vi "lstsqr_lines.vi"(8 "input error":errorcluster, 9 "weights":dbl[](array[numeric]), 10 "B points":dbl[][](array[numeric])=[[5.0, 3.0], [6.0, 6.0]], 11 "A points":dbl[][](array[numeric])=[[0.0, 1.0], [2.0, 3.0]]) -> (0 "output error":errorcluster, 3 "center":dbl[](array[numeric]))   [LabVIEW 2015]
doc: "This vi finds least square intersection point of lines defined by 2 points in arrays A and B.\nA and B are two-column arrays each containing 1 point coordiantes from each line.\nThe algorithm was adopted from \"Johannes Traa, Least-Squares Intersection of Lines, UIUC 2013\"\n\nINPUT:\nA points - 2xN array of first points that define lines (x,y)\nB points - 2xN array of second points that define lines (x,y)\nweights - 1D array\n\nOUTPUT:\ncenter - calculated least-square center of the intersection of lines\n\nAuthor: Anatolii Kashchuk"
uses:
  <vilib>/Analysis/Matrix/Datatypes/RealMatrix.ctl
  <vilib>/Utility/error.llb/Error Cluster From Error Code.vi
  <vilib>/Analysis/7linalg.llb/Solve Linear Equations (multiple right hand).vi
  <vilib>/Analysis/Matrix/Numeric/Conversions/Matrix To Array - RM.vi
  <vilib>/ErrorRing/Error Ring.xnode
  <vilib>/Analysis/NI_AALPro.lvlib
  <vilib>/Analysis/Matrix/NI_Matrix.lvlib
panel:
  out "Solution Matrix":T1
  out "q":T1
  out "R":T1
  out "XY Graph":cluster{dbl[], dbl[]}[](graph)
  # "Author: Anatolii Kashchuk"
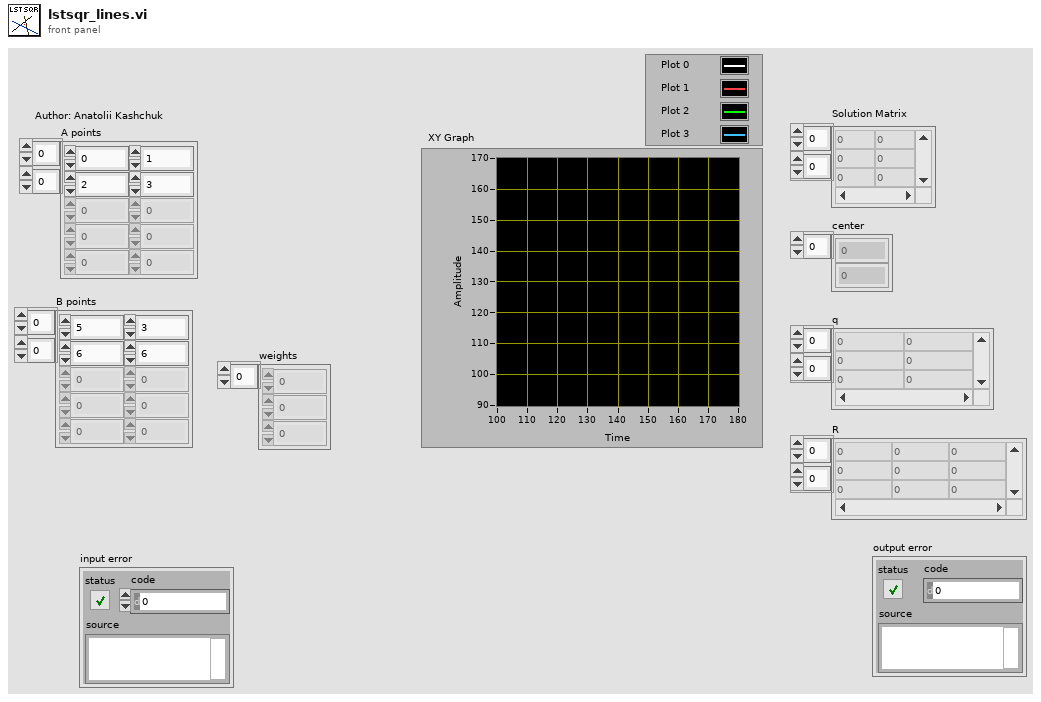
[diagram p1: front panel]
types:
  T1 = typedef "NI_Matrix.lvlib/RealMatrix.ctl" = dbl[][]
  T2 = cluster{"Real 2D Array":dbl[], "Real 2D Array":dbl[]}
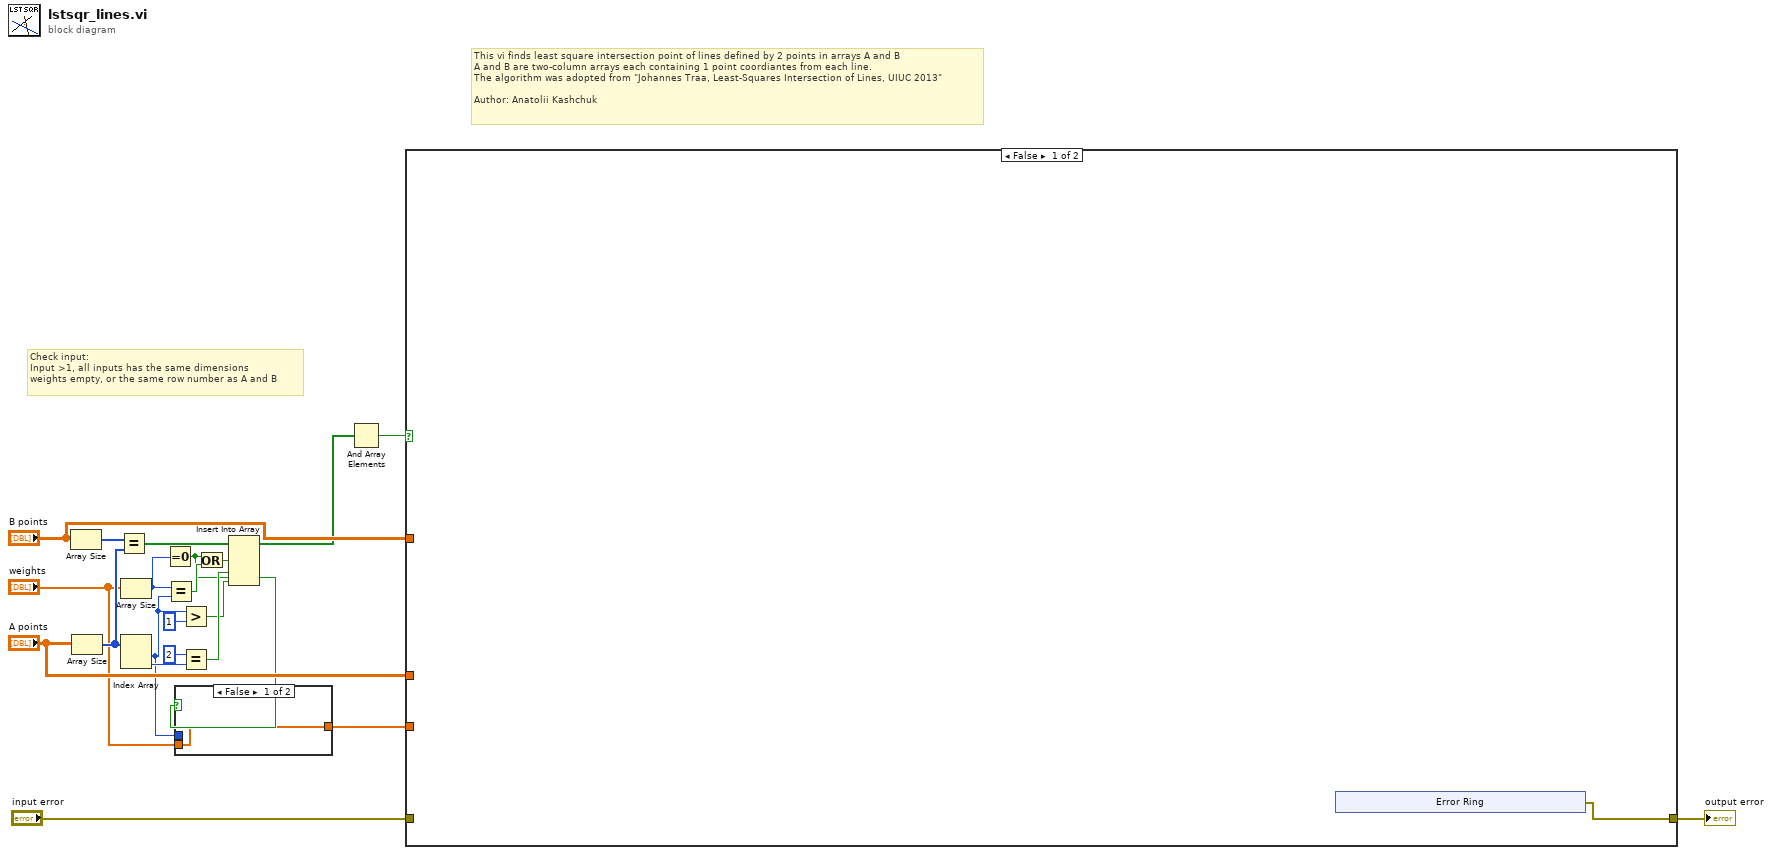
[diagram p0: block diagram]
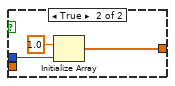
[diagram p2: hidden frame]
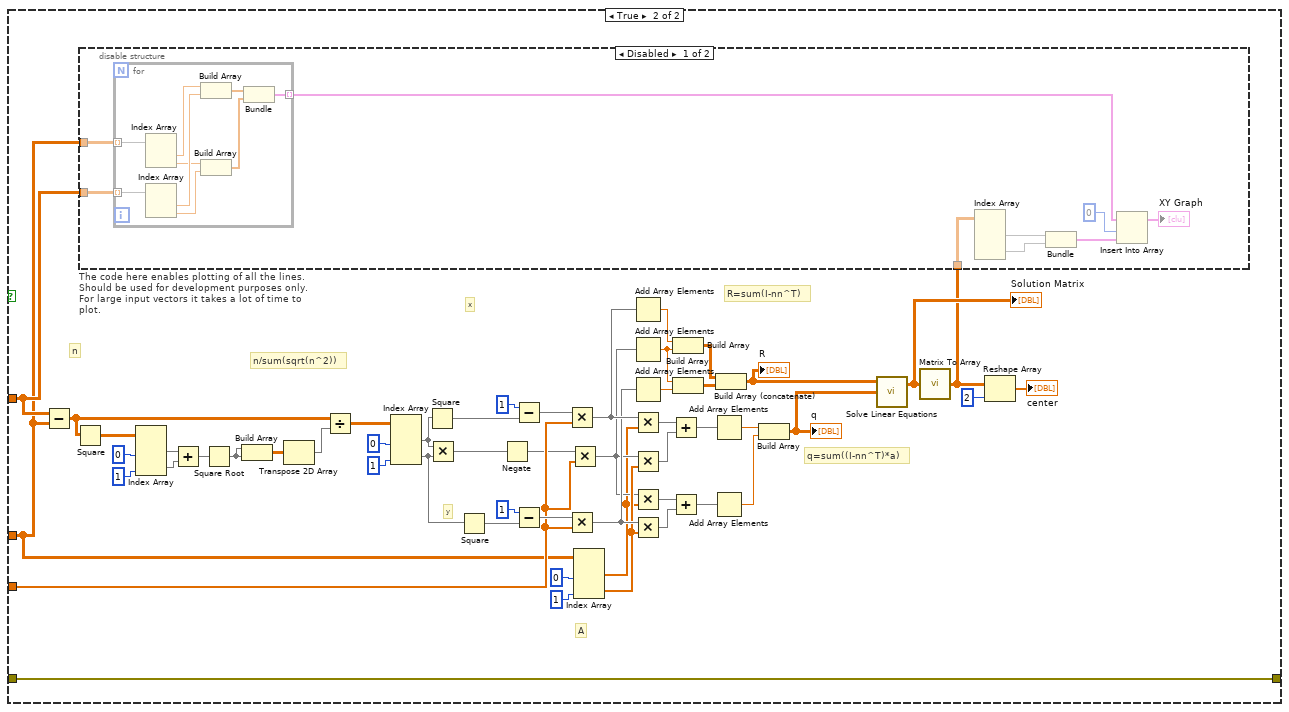
[diagram p3: hidden frame]
diagram:
  # "Check input:\nInput >1, all inputs has the same dimensions\nweights empty, or the same row number as A and B"
  # "This vi finds least square intersection point of lines defined by 2 points in arrays A and B\nA and B are two-column arrays each containing 1 point coordiantes from each line.\nThe algorithm was adopted from \"Johannes Traa, Least-Squares Intersection of Lines, UIUC 2013\"\n\nAuthor: Anatolii Kashchuk"
  n1 = Array Size(array="B points") -> (size(s)=w18:i32[])
  n2 = Array Size(array="A points") -> (size(s)=w17:i32[])
  n3 = Equal?(x=w18, y=w17) -> (x = y?=w14:bool[])
  n4 = Array Size(array="weights") -> (size(s)=w7:i32)
  n5 = Index Array(array=w17) -> (element #1=w4:i32, element #2=w16:i32)  [unwired: 2 in]
  n6 = Equal To 0?(x=w7) -> (x = 0?=w1:bool)
  n7 = Equal?(x=w7, y=w4) -> (x = y?=w6:bool)
  n8 = case shown="False" w1 {
    tunnel: w4 -> [_ w24]
    tunnel: [w22 w23] -> w3
    tunnel: "weights" -> [w22 _]
    frame False {
    }
    frame True {
      n9 = Initialize Array(1.0 ("element"), w24) -> (w23:dbl[])
    }
  }
  n10 = Greater?(x=w4, y=1) -> (0:w11:bool)
  n11 = Equal?(x=2, y=w16) -> (x = y?=w12:bool)
  n12 = Or(x=w1, y=w6) -> (x .or. y?=w5:bool)
  n13 = Insert Into Array(array=w14, new element #1=w5, new element #2=w12, new element #3=w11) -> (w13:bool[])  [unwired: 1 in]
  n14 = And Array Elements(Boolean array=w13) -> (logical AND=w19:bool)
  n15 = case shown="False" w19 {
    tunnel: w3 -> [_ w58]
    tunnel: "A points" -> [_ w49]
    tunnel: "B points" -> [_ w76]
    tunnel: "input error" -> [_ w75]
    tunnel: [w26 w75] -> w8
    frame False {
      n16 = xnode "Error Ring"() -> ("error out"=w26:errorcluster)
    }
    frame True {
      # "A"
      # "n"
      # "y"
      # "x"
      # "q=sum((I-nn^T)*a)"
      # "R=sum(I-nn^T)"
      # "n/sum(sqrt(n^2))"
      n17 = Subtract(x=w76, y=w49) -> (x-y=w84:dbl[][])
      n18 = Square(x=w84) -> (x^2=w74:dbl[][])
      n19 = Index Array(array=w74, index (col) #1=0 ("disabled index (col)"), index (col) #2=1 ("index (col)")) -> (element #1=w71:dbl[], element #2=w70:dbl[])  [unwired: 2 in]
      n20 = Add(x=w71, y=w70) -> (x+y=w69:dbl[])
      n21 = Square Root(x=w69) -> (sqrt(x)=w83:dbl[])
      n22 = Build Array(w83, w83) -> (w82:dbl[][])
      n23 = Transpose 2D Array(2D array=w82) -> (transposed array=w81:dbl[][])
      n24 = Divide(x=w84, y=w81) -> (x/y=w68:dbl[][])
      n25 = Index Array(array=w68, index (col) #1=0 ("disabled index (col)"), index (col) #2=1 ("index (col)")) -> (element #1=w65:dbl[], element #2=w64:dbl[])  [unwired: 2 in]
      n26 = Square(x=w65) -> (x^2=w63:dbl[])
      n27 = Multiply(x=w65, y=w64) -> (x*y=w57:dbl[])
      n28 = Square(x=w64) -> (x^2=w56:dbl[])
      n29 = Negate(x=w57) -> (-x=w55:dbl[])
      n30 = Subtract(x=1, y=w63) -> (x-y=w60:dbl[])
      n31 = Subtract(x=1, y=w56) -> (x-y=w59:dbl[])
      n32 = Multiply(x=w60, y=w58) -> (x*y=w46:dbl[])
      n33 = Multiply(x=w59, y=w58) -> (x*y=w42:dbl[])
      n34 = Multiply(x=w55, y=w58) -> (x*y=w37:dbl[])
      n35 = Index Array(array=w49, index (col) #1=0 ("disabled index (col)"), index (col) #2=1 ("index (col)")) -> (element #1=w36:dbl[], element #2=w41:dbl[])  [unwired: 2 in]
      n36 = Add Array Elements(numeric array=w46) -> (sum=w54:dbl)
      n37 = Add Array Elements(numeric array=w37) -> (sum=w53:dbl)
      n38 = Add Array Elements(numeric array=w42) -> (sum=w52:dbl)
      n39 = Multiply(x=w46, y=w36) -> (x*y=w45:dbl[])
      n40 = Multiply(x=w37, y=w41) -> (x*y=w39:dbl[])
      n41 = Multiply(x=w37, y=w36) -> (x*y=w38:dbl[])
      n42 = Multiply(x=w42, y=w41) -> (x*y=w40:dbl[])
      n43 = Add(x=w45, y=w39) -> (x+y=w44:dbl[])
      n44 = Add(x=w38, y=w40) -> (x+y=w43:dbl[])
      n45 = Build Array(w54, w53) -> (w50:T1)
      n46 = Build Array(w53, w52) -> (w51:T1)
      n47 = Add Array Elements(numeric array=w44) -> (sum=w35:dbl)
      n48 = Add Array Elements(numeric array=w43) -> (sum=w34:dbl)
      n49 = Build Array (concatenate)(w50, w51) -> (w33:T1)
      "R" <- w33
      n50 = Build Array(w35, w34) -> (w32:T1)
      "q" <- w32
      n51 = call-poly <vilib>:"Solve Linear Equations.vi"("Known Matrix"=w32, "Input Matrix"=w33) -> ("Solution Matrix"=w80:T1)  [unwired: 1 in, 1 out]
      "Solution Matrix" <- w80
      n52 = call-poly <vilib>:"Matrix To Array.vi"("Real Matrix"=w80) -> ("Real 2D Array"=w79:dbl[][])
      n53 = disable-structure "The code here enables plotting of all the lines. Should be used for development purposes only. For large input vectors it takes a lot of time to plot." shown="Disabled" {
        disable-tunnel: w76 -> [w93 _]
        disable-tunnel: w49 -> [w92 _]
        disable-tunnel: w79 -> [w85 _]
        frame Disabled {
          n54 = for {
            tunnel: w92 -> [w102] mode=indexing
            tunnel: w93 -> [w101] mode=indexing
            tunnel: [w94] -> w89 mode=indexing
            n55 = Index Array(array=w102) -> (element #1=w100:dbl, element #2=w97:dbl)  [unwired: 2 in]
            n56 = Index Array(array=w101) -> (element #1=w99:dbl, element #2=w96:dbl)  [unwired: 2 in]
            n57 = Build Array(w100, w99) -> (w98:dbl[])
            n58 = Build Array(w97, w96) -> (w95:dbl[])
            n59 = Bundle(w98, w95) -> (w94:cluster{dbl[], dbl[]})  [unwired: 1 in]
          }
          n60 = Index Array(array=w85) -> (element #1=w91:dbl[], element #2=w90:dbl[])  [unwired: 4 in]
          n61 = Bundle("Real 2D Array"=w91, "Real 2D Array"=w90) -> (w88:T2)  [unwired: 1 in]
          n62 = Insert Into Array(array=w89, index=0, new element=w88) -> (→"XY Graph":cluster{dbl[], dbl[]}[])
        }
        frame Enabled {
        }
      }
      n63 = Reshape Array(w79, 2 ("dimension size")) -> (→"center":dbl[])
    }
  }
  "output error" <- w8
